vi "Read Write_Dashboard to RIO controls.vi"(10 "Read(F) Write(T)":bool, 11 "Data In":T1) -> (3 "Data Out":T1)   [LabVIEW 2017]
uses:
  TypeDefs/Cluster_DashBoard to Rio Controls.ctl
  TypeDefs/ENUM_Auto Select.ctl
  <vilib>/Rock Robotics/Network Tables/NT Read Number.vi
  <vilib>/Rock Robotics/Network Tables/NT Write Number.vi
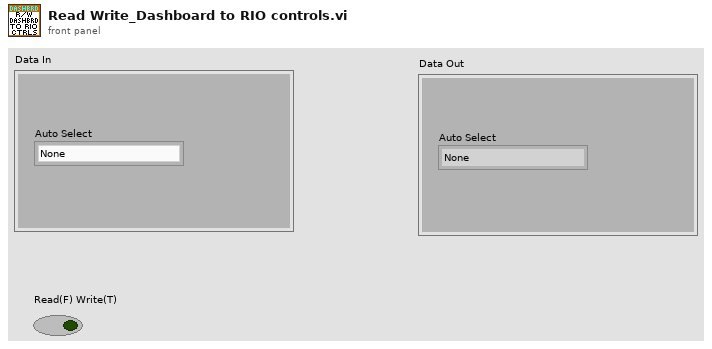
[diagram p1: front panel]
types:
  T1 = typedef "Cluster_DashBoard to Rio Controls.ctl" = cluster{"Auto Select":T2}
  T2 = typedef "ENUM_Auto Select.ctl" = enum16{"None", "Cross Baseline", "Shoot", "Middle Peg", "Right Peg", "Left Peg", "Middle Peg and Shoot", "Side Peg and Shoot", "Dump Hopper and Shoot"}
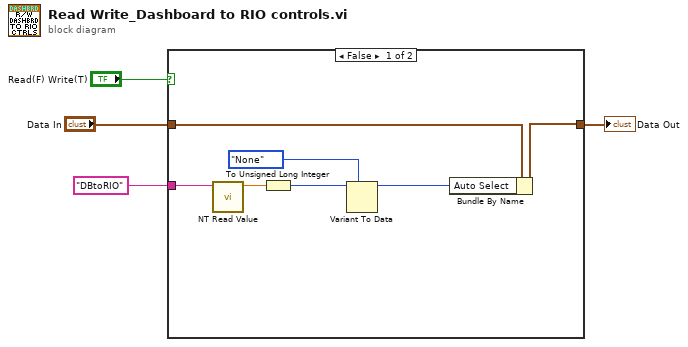
[diagram p0: block diagram]
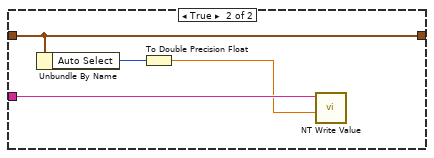
[diagram p2: hidden frame]
diagram:
  n1 = case shown="False" "Read(F) Write(T)" {
    tunnel: [w10 w15] -> w3
    tunnel: "Data In" -> [w11 w15]
    tunnel: "DBtoRIO" ("string") -> [w9 w14]
    frame False {
      n2 = call-poly <vilib>:"NT Read Value.vi"("Name"=w9) -> ("Numeric"=w8:dbl)  [unwired: 9 in, 1 out]
      n3 = To Unsigned Long Integer(number=w8) -> (unsigned 32bit integer=w7:u32)
      n4 = Variant To Data(type=ENUM_Auto_Select."None" ("Auto Setting"), Variant=w7) -> (data=w5:T2)  [unwired: 1 in, 1 out]
      n5 = Bundle By Name(cluster=w11, "Auto Select"=w5) -> (w10:T1)
    }
    frame True {
      n6 = Unbundle By Name(w15) -> ("Auto Select"=w13:T2)
      n7 = To Double Precision Float(number=w13) -> (double precision float=w12:dbl)
      n8 = call-poly <vilib>:"NT Write Value.vi"("Numeric"=w12, "Name"=w14) -> ()  [unwired: 9 in, 1 out]
    }
  }
  "Data Out" <- w3
